vi "Update Pin Information.vi"(7 "Session Reservation":refnum<class "Session Reservation.lvclass">, 8 "error in":errorcluster, 9 "channel":string, 10 "pin_name":string, 11 "instrument object in":refnum<class "DMM_Base.lvclass">) -> (0 "error out":errorcluster, 3 "instrument object out":refnum<class "DMM_Base.lvclass">)   [LabVIEW 2021, in "DMM_Base.lvclass"]
uses:
  DMM_Base.lvclass
  <vilib>/Plug-In SDKs/Clients/Session Management V1/Session Reservation/Session Reservation.lvclass
  DMM_Base.lvclass/DMM_Base.ctl
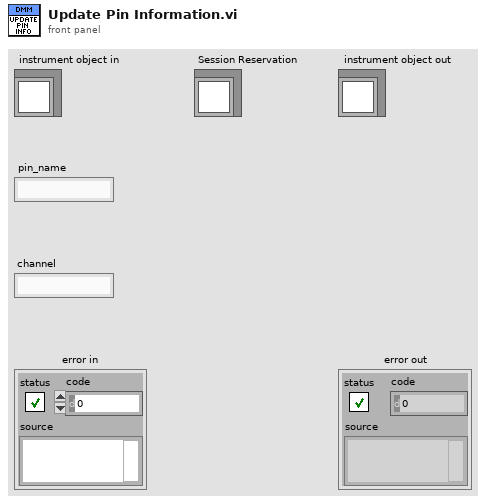
[diagram p1: front panel]
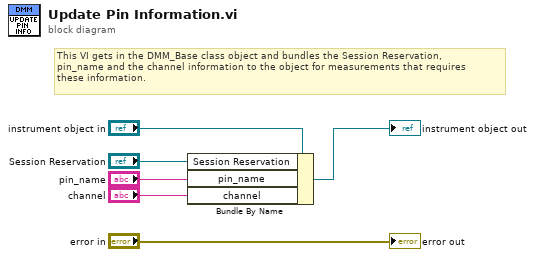
[diagram p0: block diagram]
diagram:
  # "This VI gets in the DMM_Base class object and bundles the Session Reservation,\npin_name and the channel information to the object for measurements that requires \nthese information."
  n1 = Bundle By Name(cluster="instrument object in", "Session Reservation"="Session Reservation", "pin_name"="pin_name", "channel"="channel") -> (→"instrument object out":refnum<class "DMM_Base.lvclass">)
  "error out" <- "error in"
